vi "SerialPortSetup.vi"(8 "error in (no error)":errorcluster, 10 "Serial Port Setting":T1={"stop bits "=10, "flow control (0:none)"=0, "parity (none)"=enum."None", "data bits (8)"=8, "termination char (LF)"=10, "baud rate"=19200, "resource name"="COM3", "timeout (ms)"=200} {"baud rate" items=["110"=110, "300"=300, "600"=600, "1200"=1200, "2400"=2400, "4800"=4800, "9600"=9600, "19200"=19200, "38400"=38400, "57600"=57600, "115200"=115200, "230400"=230400, "460800"=460800, "921600"=921600, "1000000"=1000000, "2000000"=2000000, "4000000"=4000000]; "termination char (LF)" format="%02x"; "data bits (8)" min=5 max=8 step=1; "flow control (0:none)" items=["None", "XON/XOFF", "RTS/CTS", "XON/XOFF & RTS/CTS", "DTR/DSR", "XON/XOFF & DTR/DSR"]; "stop bits" items=["1.0"=10, "1.5"=15, "2.0"=20]}, 11 "VISA resource name (will be closed)":refnum<visa-resource-name>) -> (0 "error out":errorcluster, 3 "VISA resource name out":refnum<visa-resource-name>)   [LabVIEW 2020]
uses:
  <vilib>/Instr/_visa.llb/VISA Configure Serial Port (Instr).vi
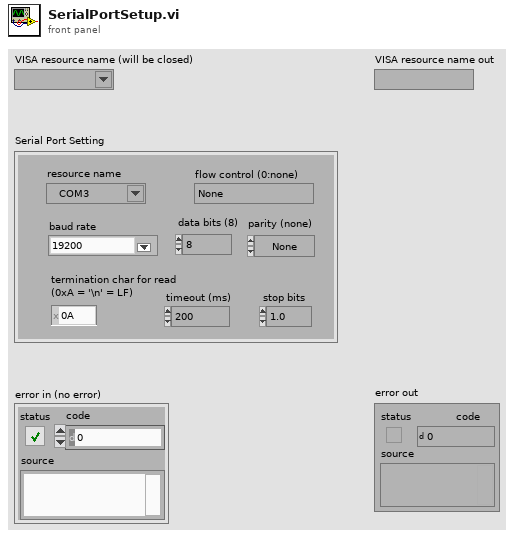
[diagram p1: front panel]
types:
  T1 = cluster{"stop bits ":u16, "flow control (0:none)":u16, "parity (none)":enum16{"None", "Odd", "Even", "Mark", "Space"}, "data bits (8)":u16, "termination char (LF)":u8, "baud rate":u32, "resource name":refnum<visa-resource-name>, "timeout (ms)":u32}
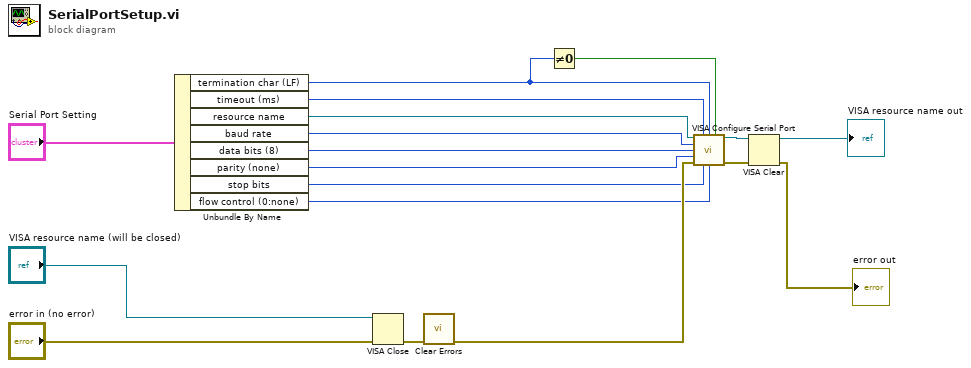
[diagram p0: block diagram]
diagram:
  n1 = Unbundle By Name("Serial Port Setting") -> ("termination char (LF)"=w5:u8, "timeout (ms)"=w12:u32, "resource name"=w10:refnum<visa-resource-name>, "baud rate"=w8:u32, "data bits (8)"=w7:u16, "parity (none)"=w6:enum16{"None", "Odd", "Even", "Mark", "Space"}, "stop bits"=w11:u16, "flow control (0:none)"=w9:u16)
  n2 = VISA Close(VISA resource name="VISA resource name (will be closed)", error in (no error)="error in (no error)") -> (error out=w15:errorcluster)
  n3 = call <vilib>:"Clear Errors.vi"("error in (no error)"=w15) -> ("error out"=w14:errorcluster)  [unwired: 5 in, 1 out]
  n4 = Not Equal To 0?(x=w5) -> (x != 0?=w4:bool)
  n5 = call-poly "VISA Configure Serial Port"("VISA resource name"=w10, "timeout (10sec)"=w12, "termination char\n(0xA = '\\n' = LF)"=w5, "Enable Termination\nChar (T)"=w4, "baud rate (9600)"=w8, "data bits (8)"=w7, "parity (0:none)"=w6, "error in (no error)"=w14, "stop bits (10: 1 bit)"=w11, "flow control (0:none)"=w9) -> ("VISA resource name out"=w17:refnum<visa-resource-name>, "error out"=w2:errorcluster)  [unwired: 4 in]
  n6 = VISA Clear(VISA resource name=w17, error in (no error)=w2) -> (VISA resource name out=→"VISA resource name out":refnum<visa-resource-name>, error out=→"error out":errorcluster)
